vi "User Plugin.vi"(5 "Initialize":bool, 8 "error in (no error)":errorcluster, 10 "ParamValues":sgl[](array[numeric]), 11 "DSI Reference":refnum<class "DCM-DSI-UserAsyncExample.lvclass">) -> (0 "error out":errorcluster, 3 "DSI Reference":refnum<class "DCM-DSI-UserAsyncExample.lvclass">, 4 "Results":T1[](array[typedef]), 6 "ParamNames":string[](array[string]))   [LabVIEW 2016, in "DCM-DSI-UserAsyncExample.lvclass"]
uses:
  DCM-DSI-UserAsyncExample.lvclass
  D:/PCG/Products/DCM/Software/DCM-DSI/Classes/DCM-DSI/DCM-DSI.lvclass
  Shared/Typedefs/UserParameter.ctl
  Vehicle Model Example/Globals/Parameter - Supra.vi
  Vehicle Model Example/Globals/Parameters - Corolla.vi
  DCM-DSI/Read Channels.vi
  DCM-DSI/Read dt.vi
  DCM-DSI/Write Channels.vi
  Shared/DSI-Shared.lvlib
  <vilib>/addons/Software Calibration Management/xSCM/SCM-API.lvlib
  Vehicle Model Example/NI-PCG Vehicle Model.lvlib
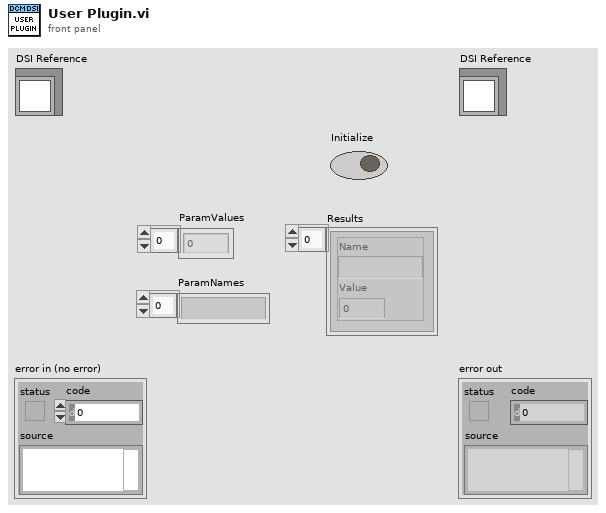
[diagram p1: front panel]
types:
  T1 = typedef "DSI-Shared.lvlib/UserParameter.ctl" = cluster{"Name":string, "Value":dbl}
  T2 = typedef "DSI-Shared.lvlib/Engine-Channel.ctl" = cluster{"Name":string, "Unit":string, "Value":sgl}
  T3 = typedef "NI-PCG Vehicle Model.lvlib/Engine Parameters.ctl" = cluster{"Ambient Parameters":cluster{"Temperature (K)":sgl, "Pressure (Pa)":sgl}, "Air Parameters":cluster{"R (Ideal Gas Constant)":sgl, "Molecular Weight":sgl, "Cp (Specific Heat Constant)":sgl, "Density (kg/m^3)":sgl, "Stoichiometric A/F Ratio":sgl}, "Engine Geometry Parameters":cluster{"Cylinder Volume (l)":sgl, "J (Rotational Moment of Inertia)":sgl, "Minimuim Engine Speed":sgl, "Maximum Engine Speed":sgl, "Intake Manifold Volume (l)":sgl}, "Volumetric Efficiency Map":cluster{"MAP":sgl[], "RPM":sgl[], "Table":sgl[][]}, "Fuel LHV (J/kg)":sgl, "Combustion Efficiency Map":cluster{"Spark Timing (deg BTDC))":sgl[], "Engine Speed (RPM)":sgl[], "Combustion Efficiency":sgl[][]}, "Thermodynamic Efficiency":sgl}
  T4 = typedef "NI-PCG Vehicle Model.lvlib/Transmission Parameters.ctl" = cluster{"Final Drive Ratio":sgl, "Transmission Gear Ratios":cluster{"Gears":sgl[], "Gear Ratios":sgl[]}, "Torque Converter Map":cluster{"Speed Ratio":sgl[], "K Factor":sgl[], "Torque Ratio":sgl[]}, "Upshift Throttle":sgl[], "Downshift Throttle":sgl[], "Upshift Table":sgl[][], "Downshift Table":sgl[][], "Wait Time":u8}
  T5 = typedef "NI-PCG Vehicle Model.lvlib/Vehicle Parameters.ctl" = cluster{"Vehicle Mass (kg)":sgl, "Vehicle Cd":sgl, "Vehicle Frontal Area (m^2)":sgl, "Wheel Radius (m)":sgl, "Wheel Rolling Resistance":sgl}
  T6 = cluster{"Engine Parameters":T3, "Transmission Parameters":T4, "Vehicle Parameters":T5}
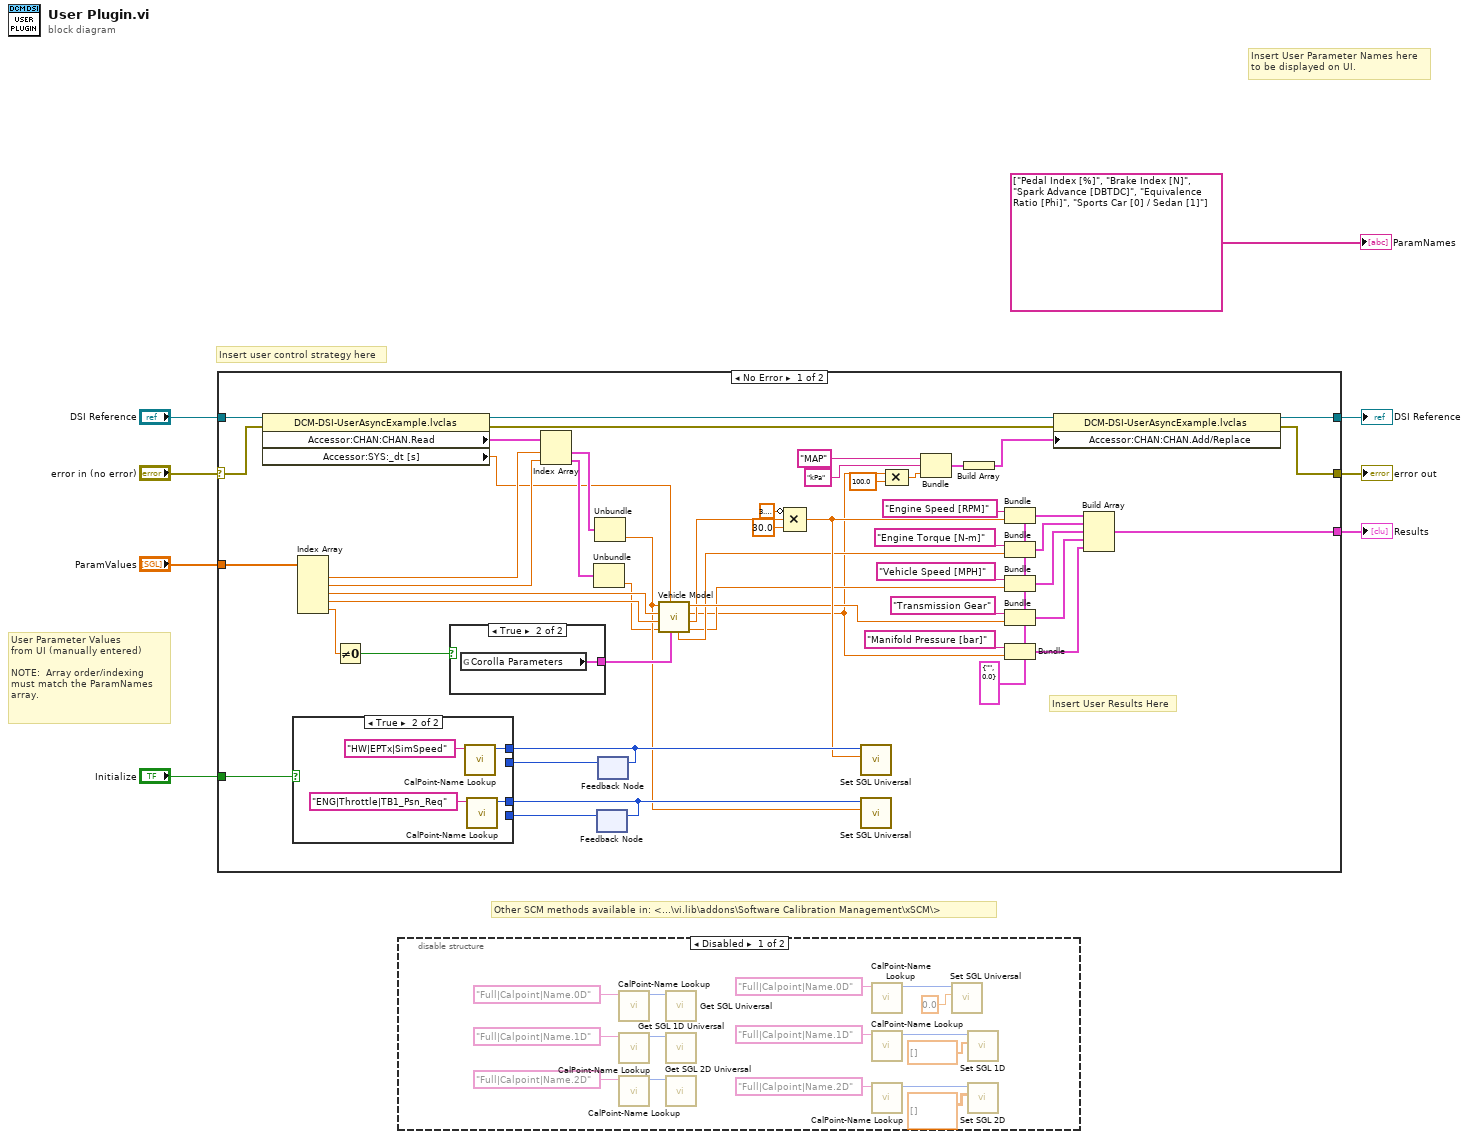
[diagram p0: block diagram]
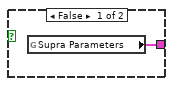
[diagram p4: hidden frame]
diagram:
  # "Other SCM methods available in: <...\\vi.lib\\addons\\Software Calibration Management\\xSCM\\>"
  # "User Parameter Values\nfrom UI (manually entered)\n\nNOTE:  Array order/indexing\nmust match the ParamNames\narray."
  # "Insert user control strategy here"
  # "Insert User Parameter Names here\nto be displayed on UI."
  n1 = case shown="No Error" "error in (no error)" {
    selector: "error in (no error)" -> [w59 w69]
    tunnel: [w18 w69] -> w7
    tunnel: [w19 w68] -> w5
    tunnel: "DSI Reference" -> [w58 w68]
    tunnel: "Initialize" -> [w36 _]
    tunnel: "ParamValues" -> [w38 _]
    tunnel: [w37 _] -> w2
    frame No Error {
      w39 = T1 {"Name"="", "Value"=0.0} ("User Parameter")
      # "Insert User Results Here"
      n2 = property class="DCM-DSI-UserAsyncExample.lvclas"(reference=w58, error in=w59) -> (reference out=w21:refnum<class "DCM-DSI-UserAsyncExample.lvclass">, error out=w20:errorcluster, "Accessor:CHAN:CHAN.Read"=w16:T2[], "Accessor:SYS:_dt [s]"=w17:sgl)
      n3 = Index Array(array=w38) -> (element #1=w28:sgl, element #2=w27:sgl, element #3=w34:sgl, element #4=w35:sgl, element #5=w23:sgl)  [unwired: 5 in]
      n4 = Not Equal To 0?(x=w23) -> (x != 0?=w52:bool)
      n5 = case shown="True" w52 {
        tunnel: [w66 w67] -> w32
        frame False {
          n6 = global read "Parameter - Supra.vi" "Supra Parameters"() -> (w66:T6)
        }
        frame True {
          n7 = global read "Parameters - Corolla.vi" "Corolla Parameters"() -> (w67:T6)
        }
      }
      n8 = Index Array(array=w16, index #1=w28, index #2=w27) -> (element #1=w26:T2, element #2=w25:T2)
      n9 = Unbundle(w25) -> ("Value"=w22:sgl)  [unwired: 2 out]
      n10 = Unbundle(w26) -> ("Value"=w24:sgl)  [unwired: 2 out]
      n11 = feedback #1() -> (w57:u32)  [unwired: 1 in]
      n12 = feedback #2() -> (w56:u32)  [unwired: 1 in]
      n13 = case shown="True" w36 {
        tunnel: [w61 w64] -> w55
        tunnel: [w60 w63] -> w54
        tunnel: w56 -> [w61 _]
        tunnel: w57 -> [w60 _]
        frame False {
        }
        frame True {
          n14 = call <vilib>:"CalPoint-Name Lookup.vi"("Name"="HW|EPTx|SimSpeed") -> ("ID"=w64:u32)  [unwired: 9 in, 1 out]
          n15 = call <vilib>:"CalPoint-Name Lookup.vi"("Name"="ENG|Throttle|TB1_Psn_Req") -> ("ID"=w63:u32)  [unwired: 9 in, 1 out]
        }
      }
      n16 = feedback-in #1(w54) -> ()
      n17 = feedback-in #2(w55) -> ()
      n18 = call "Vehicle Model.vi"("Parameters"=w32, "dt"=w17, "Brake Force (N)"=w22, "phi"=w35, "Spark Advance (deg BTDC)"=w34, "Throttle Angle (deg)"=w24) -> ("Vehicle Speed (miles per hour)"=w30:sgl, "Engine Speed (rad/s)"=w29:sgl, "Manifold Pressure (bar)"=w12:sgl, "Gear"=w33:sgl, "EngineTorque (N-m)"=w31:sgl)  [unwired: 1 in]
      n19 = Compound Arithmetic op=MULTIPLY(invert 3.141592653589793, w29, sgl 30.0 ("value")) -> (w53:dbl)
      n20 = call <vilib>:"Set SGL Universal.vi"("Data"=w53, "ID"=w55) -> ()  [unwired: 10 in]
      n21 = call <vilib>:"Set SGL Universal.vi"("Data"=w24, "ID"=w54) -> ()  [unwired: 10 in]
      n22 = Compound Arithmetic op=MULTIPLY(w12, sgl 100.0 ("value")) -> (w11:sgl)
      n23 = Bundle("Name"="MAP", "Name"="kPa", w11) -> (w13:cluster{"Name":string, "Name":string, sgl})  [unwired: 1 in]
      n24 = Build Array(w13) -> (w9:cluster{"Name":string, "Name":string, sgl}[])
      n25 = Bundle(cluster=w39, "Name"="Engine Speed [RPM]", "Value"=w53) -> (w45:T1)
      n26 = Bundle(cluster=w39, "Name"="Engine Torque [N-m]", "Value"=w31) -> (w46:T1)
      n27 = Bundle(cluster=w39, "Name"="Vehicle Speed [MPH]", "Value"=w30) -> (w47:T1)
      n28 = Bundle(cluster=w39, "Name"="Transmission Gear", "Value"=w33) -> (w48:T1)
      n29 = Bundle(cluster=w39, "Name"="Manifold Pressure [bar]", "Value"=w12) -> (w49:T1)
      n30 = property class="DCM-DSI-UserAsyncExample.lvclas"(reference=w21, error in=w20, "Accessor:CHAN:CHAN.Add/Replace"=w9) -> (reference out=w19:refnum<class "DCM-DSI-UserAsyncExample.lvclass">, error out=w18:errorcluster)
      n31 = Build Array(w45, w46, w47, w48, w49) -> (w37:T1[])
    }
    frame Error {
    }
  }
  "error out" <- w7
  "DSI Reference" <- w5
  "Results" <- w2
  n32 = disable-structure shown="Disabled" {
    frame Disabled {
      n33 = call <vilib>:"CalPoint-Name Lookup.vi"("Name"="Full|Calpoint|Name.0D") -> ("ID"=w79:u32)  [unwired: 9 in, 1 out]
      n34 = call <vilib>:"CalPoint-Name Lookup.vi"("Name"="Full|Calpoint|Name.1D") -> ("ID"=w78:u32)  [unwired: 9 in, 1 out]
      n35 = call <vilib>:"CalPoint-Name Lookup.vi"("Name"="Full|Calpoint|Name.2D") -> ("ID"=w76:u32)  [unwired: 9 in, 1 out]
      n36 = call <vilib>:"Get SGL Universal.vi"("ID"=w79) -> ()  [unwired: 10 in, 1 out]
      n37 = call <vilib>:"Get SGL 1D Universal.vi"("ID"=w78) -> ()  [unwired: 10 in, 1 out]
      n38 = call <vilib>:"Get SGL 2D Universal.vi"("ID"=w76) -> ()  [unwired: 10 in, 1 out]
      n39 = call <vilib>:"CalPoint-Name Lookup.vi"("Name"="Full|Calpoint|Name.0D") -> ("ID"=w82:u32)  [unwired: 9 in, 1 out]
      n40 = call <vilib>:"CalPoint-Name Lookup.vi"("Name"="Full|Calpoint|Name.1D") -> ("ID"=w74:u32)  [unwired: 9 in, 1 out]
      n41 = call <vilib>:"CalPoint-Name Lookup.vi"("Name"="Full|Calpoint|Name.2D") -> ("ID"=w71:u32)  [unwired: 9 in, 1 out]
      n42 = call <vilib>:"Set SGL Universal.vi"("Data"=sgl 0.0 ("Value"), "ID"=w82) -> ()  [unwired: 10 in]
      n43 = call <vilib>:"Set SGL 1D.vi"("Data"=sgl[] [] ("Value"), "ID"=w74) -> ()  [unwired: 10 in]
      n44 = call <vilib>:"Set SGL 2D.vi"("Data"=sgl[][] [] ("Value"), "ID"=w71) -> ()  [unwired: 10 in]
    }
    frame Enabled {
    }
  }
  "ParamNames" <- string[] ["Pedal Index [%]", "Brake Index [N]", "Spark Advance [DBTDC]", "Equivalence Ratio [Phi]", "Sports Car [0] / Sedan [1]"]
